vi "setValue.vi"(8 "error in (no error)":errorcluster, 10 "Value":refnum<class "tBSONDocument.lvclass">, 11 "tBSONDocumentElement in":refnum<class "tBSONDocumentElement.lvclass">) -> (0 "error out":errorcluster, 3 "tBSONDocumentElement out":refnum<class "tBSONDocumentElement.lvclass">)   [LabVIEW 2013, in "BSON.lvlib" / "tBSONDocumentElement.lvclass"]
uses:
  tBSONDocumentElement.lvclass
  tBSONDocument/tBSONDocument.lvclass
  tBSONDocumentElement.lvclass/tBSONDocumentElement.ctl
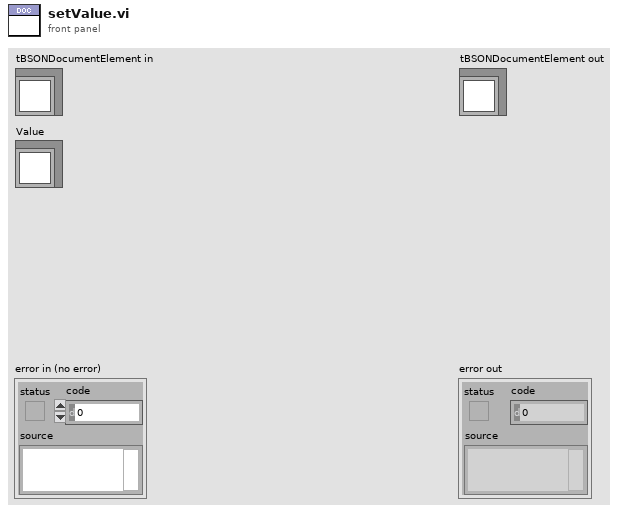
[diagram p1: front panel]
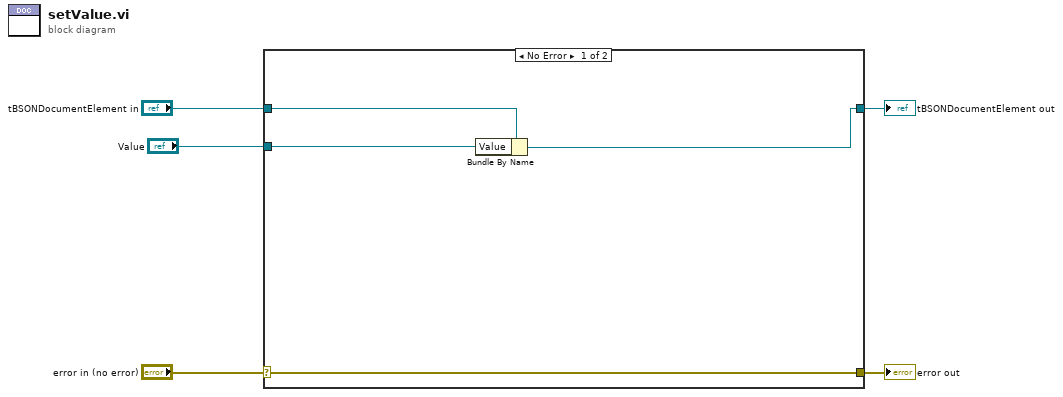
[diagram p0: block diagram]
diagram:
  n1 = case shown="No Error" "error in (no error)" {
    selector: "error in (no error)" -> [w9 w11]
    tunnel: [w9 w11] -> w4
    tunnel: [w6 w10] -> w2
    tunnel: "tBSONDocumentElement in" -> [w8 w10]
    tunnel: "Value" -> [w7 _]
    frame No Error {
      n2 = Bundle By Name(cluster=w8, "Value"=w7) -> (w6:refnum<class "tBSONDocumentElement.lvclass">)
    }
    frame Error {
    }
  }
  "error out" <- w4
  "tBSONDocumentElement out" <- w2
